vi "6.vi"() -> ()   [LabVIEW 2017]
panel:
  out "波形图":dbl[](graph)
  out "最小值":dbl
  out "最大值":dbl
  out "平均值":dbl
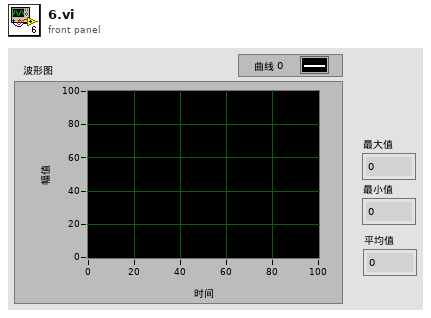
[diagram p1: front panel]
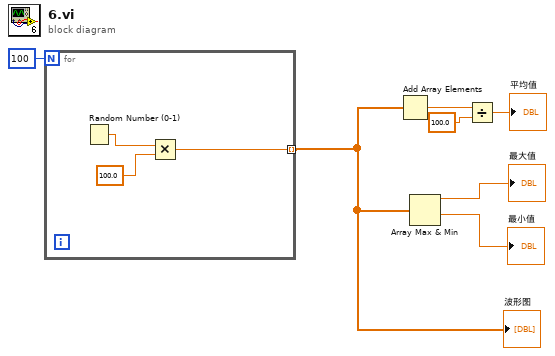
[diagram p0: block diagram]
diagram:
  n1 = for {
    N: 100 -> [_]
    tunnel: [w8] -> w1 mode=indexing
    n2 = Random Number (0-1)() -> (number: 0 to 1=w10:dbl)
    n3 = Multiply(x=w10, y=100.0) -> (x*y=w8:dbl)
  }
  "波形图" <- w1
  n4 = Add Array Elements(numeric array=w1) -> (sum=w6:dbl)
  n5 = Array Max & Min(array=w1) -> (max value=→"最大值":dbl, min value=→"最小值":dbl)  [unwired: 2 out]
  n6 = Divide(x=w6, y=100.0) -> (x/y=→"平均值":dbl)
